vi "PIDControllers.vi"() -> ()   [LabVIEW 2017]
uses:
  <vilib>/Platform/TimedLoop/XDataNode/timing_clust.ctl
  <vilib>/Platform/TimedLoop/XDataNode/nitl_modes.ctl
  <vilib>/Platform/TimedLoop/XDataNode/wakeup.ctl
  <vilib>/addons/control/pid/pid.llb/PID Advanced (DBL).vi
  <vilib>/Platform/TimedLoop/XDataNode/XDataNode.xnode
  <vilib>/Platform/TimedLoop/XDataNode/XDNodeRunTimeDep.lvlib
  <vilib>/addons/control/pid/NI_PID_pid.lvlib
panel:
  in  "stop":bool
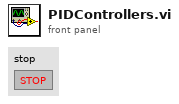
[diagram p1: front panel]
types:
  T1 = typedef "XDNodeRunTimeDep.lvlib/timing_clust.ctl" = cluster{"Expected End [f-1]":u64, "Actual End [f-1]":u64, "Finished Late? [f-1]":bool, "Expected End [i-1]":u64, "Actual End [i-1]":u64, "Finished Late? [i-1]":bool, "Expected Start [i]":u64, "Actual Start [i]":u64, "Expected Start [f]":u64, "Actual Start [f]":u64, "Source Name":string, "Structure Name":string, "Period":i64, "Deadline":i64, "Offset":i64, "Start":i64, "Priority":i32, "Timeout":i32, "Mode":T2, "Wakeup Reason":T3, "Error":errorcluster, "Source Type":string, "Secondary Source Type":string, "Global End Time":u64, "Global Start Time":u64, "Frame Duration":u64, "Iteration Duration":u64, "Assigned CPU":i32, "I/O Scan Engine Mode":u32}
  T2 = typedef "XDNodeRunTimeDep.lvlib/nitl_modes.ctl" = enum32{"No Change", "Process missed periods, maintain original phase", "Discard missed periods, maintain original phase", "Process missed periods, ignore original phase", "Discard missed periods, ignore original phase"}
  T3 = typedef "XDNodeRunTimeDep.lvlib/wakeup.ctl" = enum32{"Normal", "Aborted", "Asynchronous wakeup", "Timing source error", "Timed loop error", "Timeout"}
  T4 = cluster{"Array of Double[0]":dbl, "Array of Double[1]":dbl, "Array of Double[2]":dbl}
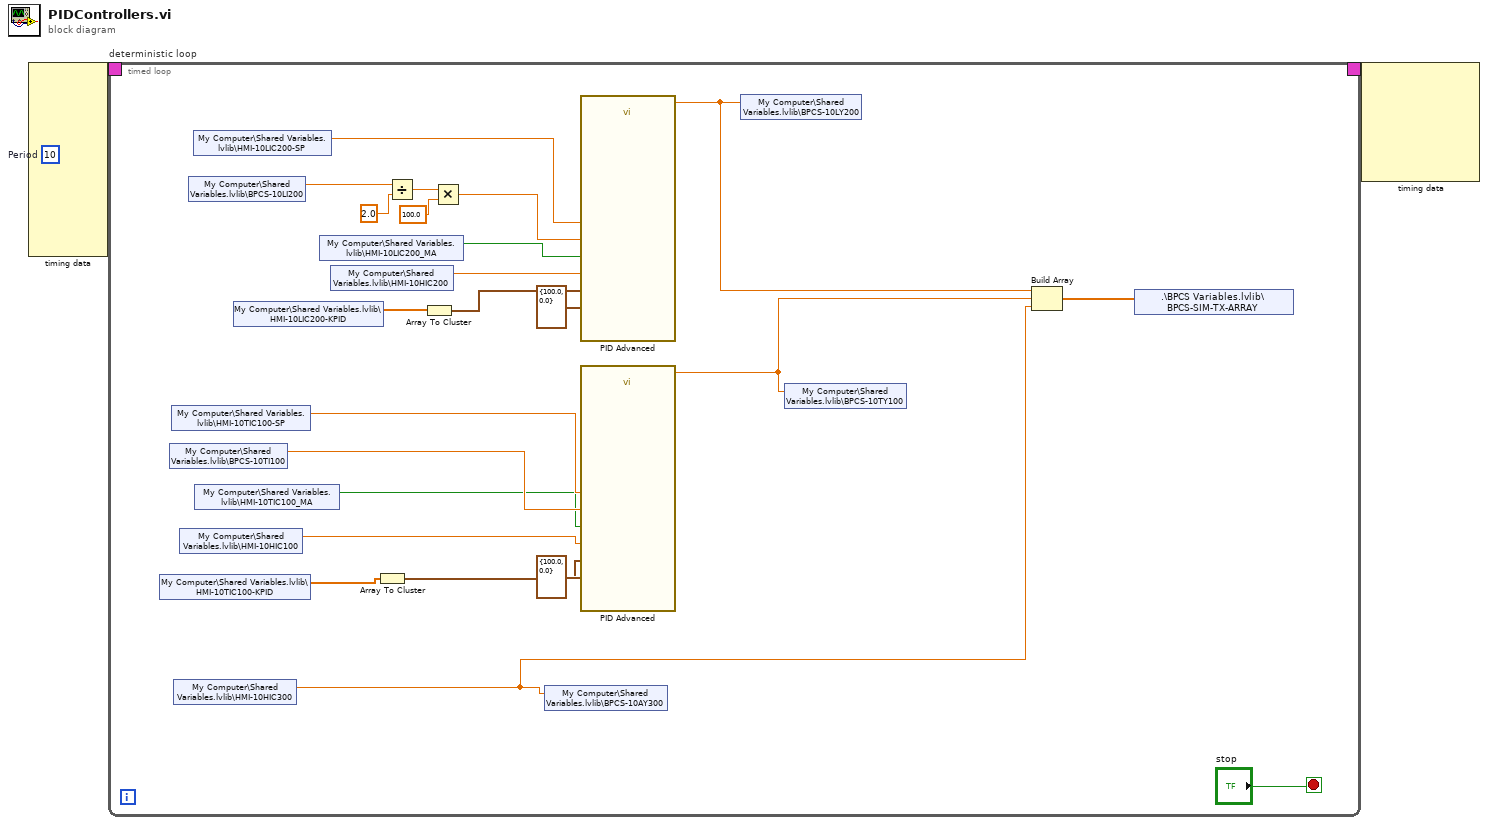
[diagram p0: block diagram]
diagram:
  w1 = i64 10  # Period
  n1 = node-c288 ("Input Node")(w1) -> (w3:T1)  [unwired: 9 in]
  n2 = timed-loop "deterministic loop" {
    timing: w3 -> [_]
    timing-out: [_] -> w2
    stop <- "stop" stop-if-true
    n3 = shared-variable "My Computer\\Shared Variables.lvlib\\HMI-10TIC100-KPID"() -> (w10:dbl[])  [unwired: 1 in, 1 out]
    n4 = shared-variable "My Computer\\Shared Variables.lvlib\\BPCS-10TI100"() -> (w13:dbl)  [unwired: 1 in, 1 out]
    n5 = shared-variable "My Computer\\Shared Variables.lvlib\\HMI-10TIC100-SP"() -> (w14:dbl)  [unwired: 1 in, 1 out]
    n6 = shared-variable "My Computer\\Shared Variables.lvlib\\HMI-10HIC300"() -> (w5:dbl)  [unwired: 1 in, 1 out]
    n7 = shared-variable "My Computer\\Shared Variables.lvlib\\HMI-10HIC100"() -> (w11:dbl)  [unwired: 1 in, 1 out]
    n8 = shared-variable "My Computer\\Shared Variables.lvlib\\BPCS-10LI200"() -> (w23:dbl)  [unwired: 1 in, 1 out]
    n9 = shared-variable "My Computer\\Shared Variables.lvlib\\HMI-10LIC200-SP"() -> (w21:dbl)  [unwired: 1 in, 1 out]
    n10 = shared-variable "My Computer\\Shared Variables.lvlib\\HMI-10TIC100_MA"() -> (w12:bool)  [unwired: 1 in, 1 out]
    n11 = shared-variable "My Computer\\Shared Variables.lvlib\\HMI-10LIC200-KPID"() -> (w22:dbl[])  [unwired: 1 in, 1 out]
    n12 = shared-variable "My Computer\\Shared Variables.lvlib\\HMI-10LIC200_MA"() -> (w17:bool)  [unwired: 1 in, 1 out]
    n13 = shared-variable "My Computer\\Shared Variables.lvlib\\HMI-10HIC200"() -> (w18:dbl)  [unwired: 1 in, 1 out]
    n14 = Array To Cluster(array=w10) -> (cluster=w9:T4)
    n15 = Divide(x=w23, y=2.0 ("x")) -> (x/y=w25:dbl)
    n16 = Array To Cluster(array=w22) -> (cluster=w19:T4)
    n17 = Multiply(x=w25, y=100.0) -> (x*y=w20:dbl)
    n18 = shared-variable "My Computer\\Shared Variables.lvlib\\BPCS-10AY300"(w5) -> ()  [unwired: 1 in, 1 out]
    n19 = call-poly <vilib>:"PID Advanced.vi"("setpoint"=w21, "output range"=cluster{"output high":dbl, "output low":dbl} {"output high"=100.0, "output low"=0.0}, "auto? (T)"=w17, "manual control"=w18, "process variable"=w20, "PID gains"=w19) -> ("output"=w7:dbl)  [unwired: 8 in, 1 out]
    n20 = call-poly <vilib>:"PID Advanced.vi"("setpoint"=w14, "output range"=cluster{"output high":dbl, "output low":dbl} {"output high"=100.0, "output low"=0.0}, "auto? (T)"=w12, "manual control"=w11, "process variable"=w13, "PID gains"=w9) -> ("output"=w6:dbl)  [unwired: 8 in, 1 out]
    n21 = shared-variable "My Computer\\Shared Variables.lvlib\\BPCS-10LY200"(w7) -> ()  [unwired: 1 in, 1 out]
    n22 = shared-variable "My Computer\\Shared Variables.lvlib\\BPCS-10TY100"(w6) -> ()  [unwired: 1 in, 1 out]
    n23 = Build Array(w7, w6, w5) -> (w4:dbl[])
    n24 = shared-variable ".\\BPCS Variables.lvlib\\BPCS-SIM-TX-ARRAY"(w4) -> ()  [unwired: 1 in, 1 out]
  }
  n25 = node-c288 ("Output Node")(w2) -> ()  [unwired: 6 out]
